vi "Enregistrement des parametres.vi"() -> ()   [LabVIEW 2011]
panel:
  out "Processing":u8(slide) scale=0.0..100.0
  # "Enregistrement des données ..."
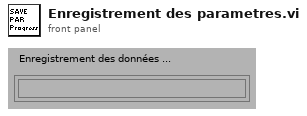
[diagram p1: front panel]
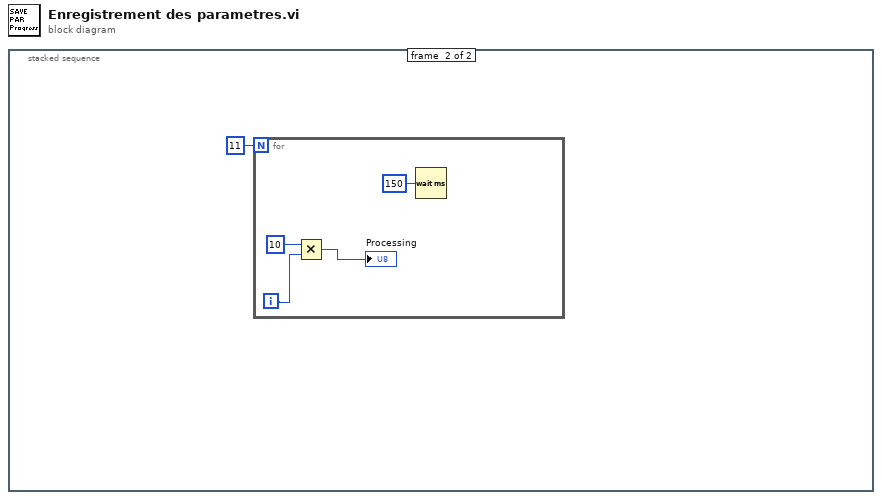
[diagram p0: block diagram]
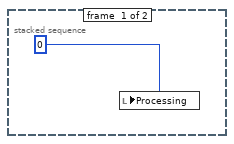
[diagram p2: hidden frame]
diagram:
  n1 = stacked-sequence {
    frame #0 {
      n2 = local write "Processing"(0) -> ()
    }
    frame #1 {
      n3 = for {
        N: 11 -> [_]
        i -> [w5]
        n4 = Multiply(x=10, y=w5) -> (x*y=→"Processing":i32)
        n5 = Wait (ms)(milliseconds to wait=u32 150 ("n millisecondes")) -> ()  [unwired: 1 out]
      }
    }
  }
